vi "Convert JSONPath to Excel Table Path.vi"(8 "error in":errorcluster, 11 "JSONPath":string) -> (0 "error out":errorcluster, 2 "Column":string, 3 "Table Name":string)   [LabVIEW 2019, in "Config from EXCEL.lvclass"]
uses:
  Config from EXCEL.lvclass
  Config from EXCEL.lvclass/Config from EXCEL.ctl
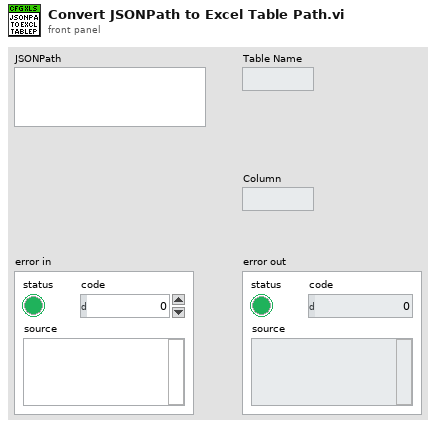
[diagram p1: front panel]
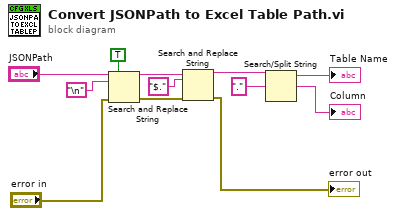
[diagram p0: block diagram]
diagram:
  n1 = Search and Replace String(replace all?=TRUE ("replace all? (F)"), input string="JSONPath", search string="\n", error in="error in") -> (result string=w7:string, error out=w5:errorcluster)  [unwired: 4 in, 2 out]
  n2 = Search and Replace String(input string=w7, search string="$." ("search string/char (-)"), error in=w5) -> (result string=w4:string, error out=→"error out":errorcluster)  [unwired: 5 in, 2 out]
  n3 = Search/Split String(string=w4, search string/char (-)="." ("Split Pattern")) -> (substring before match=→"Table Name":string, match + rest of string=→"Column":string)  [unwired: 1 in, 1 out]
